vi "Siri (SubVI).vi"(3 "error in (no error)":errorcluster, 4 "Voice Controlled Input Pin":u8, 5 "Arduino Resource in":T1) -> (0 "error out":errorcluster, 1 "Voice Command Status":bool, 2 "Arduino Resource out":T1)   [LabVIEW 2015]
uses:
  <vilib>/LabVIEW Interface for Arduino/Type Defs/Arduino Resource.ctl
  <vilib>/LabVIEW Interface for Arduino/Type Defs/Board Type.ctl
  <vilib>/LabVIEW Interface for Arduino/LabVIEW Interface for Arduino.lvlib
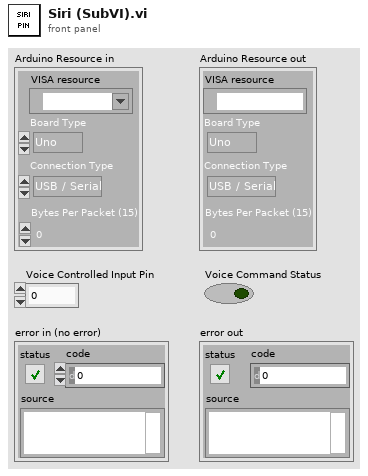
[diagram p1: front panel]
types:
  T1 = typedef "LabVIEW Interface for Arduino.lvlib/Arduino Resource.ctl" = cluster{"VISA resource":refnum<visa-resource-name>, "Board Type":T2, "Connection Type":enum8{"USB / Serial"}, "Bytes Per Packet (15)":u8}
  T2 = typedef "LabVIEW Interface for Arduino.lvlib/Board Type.ctl" = enum16{"Uno", "Dimuelanove w/Atmega 328", "Mega 2560"}
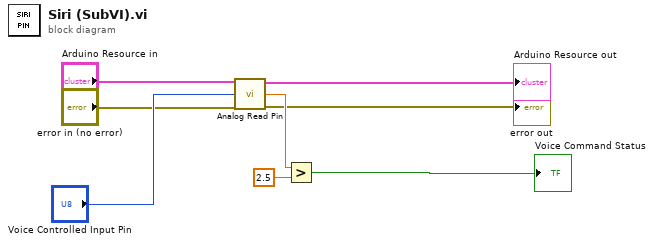
[diagram p0: block diagram]
diagram:
  n1 = call <vilib>:"Analog Read Pin.vi"("Arduino Resource"="Arduino Resource in", "Analog Input Pin (0)"="Voice Controlled Input Pin", "error in"="error in (no error)") -> ("Arduino Resource"=→"Arduino Resource out":T1, "Voltage"=w6:dbl, "error out"=→"error out":errorcluster)  [unwired: 10 in]
  n2 = Greater?(x=w6, y=2.5) -> (0:→"Voice Command Status":bool)
